vi "Cache File Entry--constant.vi"() -> (3 "Entry":string="DebugElementsCacheFile")   [LabVIEW 2020]
doc: "Entry in LabVIEW.ini where the <b>Cache File</b> location is stored."
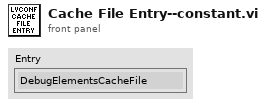
[diagram p1: front panel]
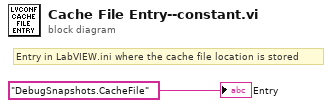
[diagram p0: block diagram]
diagram:
  # "Entry in LabVIEW.ini where the cache file location is stored"
  "Entry" <- "DebugSnapshots.CacheFile"
